vi "Measurement UI.vi"() -> ()   [LabVIEW 2021, in "Advanced Data Structure Exchange UI.lvlib"]
uses:
  Advanced Data Structure Exchange UI.lvlib
  Advanced Data Structure Exchange/Cluster In.ctl
  Advanced Data Structure Exchange/Cluster Out.ctl
  f0fe0f58-f2b4-4143-8e8a-3af1e57b7123.vi
  ddf3fbea-121e-4524-8916-c867006085d0.vi
  830132d3-c9aa-4633-b2df-af3633884cec.vi
  de374512-88bd-4d17-83f8-57bd328874a2.vi
  <vilib>/JDP Science/JSONtext/Variant to JSON Text.vi
  <vilib>/JDP Science/JSONtext/JSON text to Variant.vi
  <vilib>/JDP Science/JSONtext/LVClass Serializer/JSONtext LVClass Serializer.lvclass
  Advanced Data Structure Exchange/Advanced Data Structure Exchange.lvlib
panel:
  out "Cluster Out str":string
  in  "Cluster In str":string
  in  "Data Exchange Medium":enum32{"JSON String", "Text File"}(ring)
  in  "Text File Path":path
  out "Cluster Out":T1
  in  "Cluster In":T2 {"Text Ring" items=["Default", "Custom"]}
  # "(Choose only if Date exchange is through File)"
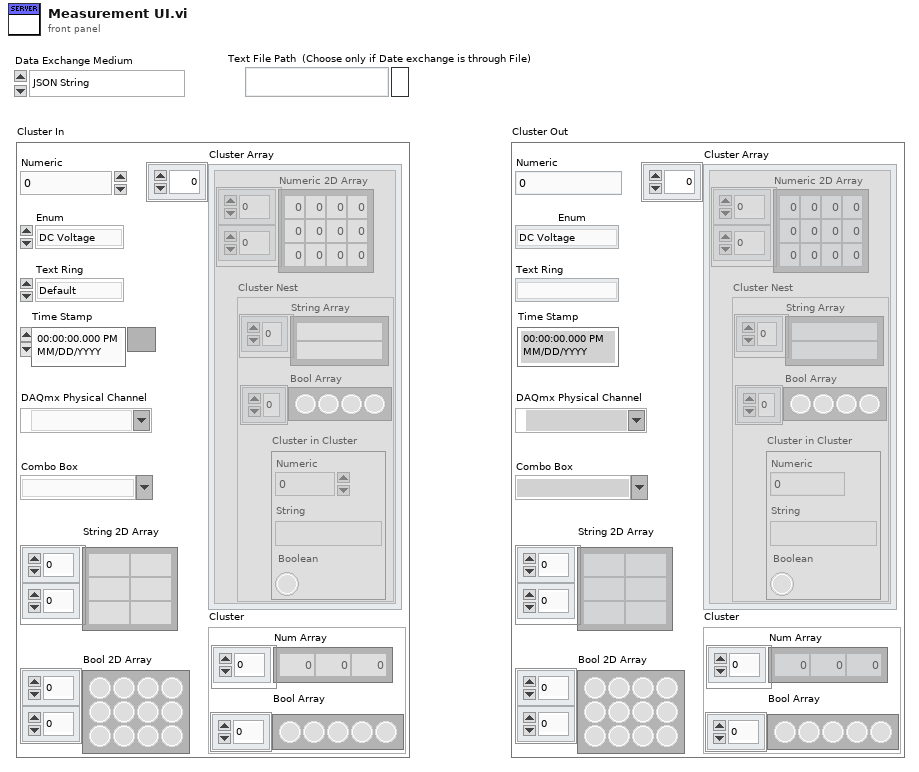
[diagram p1: front panel]
types:
  T1 = typedef "Advanced Data Structure Exchange.lvlib/Cluster Out.ctl" = cluster{"Numeric":dbl, "Bool 2D Array":bool[][], "String 2D Array":string[][], "Text Ring":u16, "Cluster":cluster{"Num Array":dbl[], "Bool Array":bool[]}, "Time Stamp":timestamp, "Enum":enum16{"DC Voltage", "DC Current"}, "DAQmx Physical Channel":tag, "Combo Box":string, "Cluster Array":cluster{"Numeric 2D Array":dbl[][], "Cluster Nest":cluster{"String Array":string[], "Bool Array":bool[], "Cluster in Cluster":cluster{"Numeric":dbl, "Boolean":bool, "String":string}}}[]}
  T2 = typedef "Advanced Data Structure Exchange.lvlib/Cluster In.ctl" = cluster{"Numeric":dbl, "Bool 2D Array":bool[][], "String 2D Array":string[][], "Text Ring":u16, "Cluster":cluster{"Num Array":dbl[], "Bool Array":bool[]}, "Time Stamp":timestamp, "Enum":enum16{"DC Voltage", "DC Current"}, "DAQmx Physical Channel":tag, "Combo Box":string, "Cluster Array":cluster{"Numeric 2D Array":dbl[][], "Cluster Nest":cluster{"String Array":string[], "Bool Array":bool[], "Cluster in Cluster":cluster{"Numeric":dbl, "Boolean":bool, "String":string}}}[]}
  T3 = enum16{"open", "replace", "create", "open or create", "replace or create", "replace or create with confirmation"}
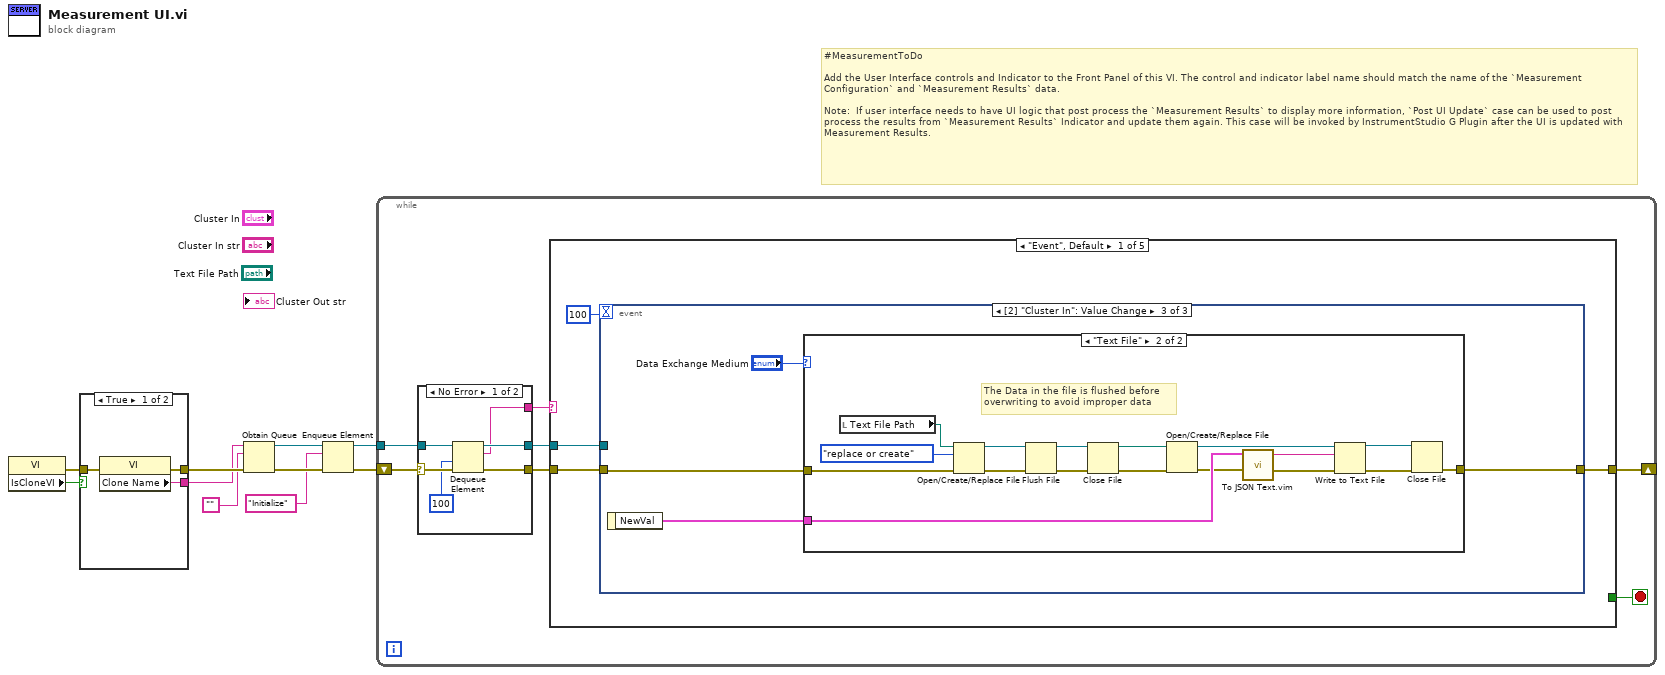
[diagram p0: block diagram]
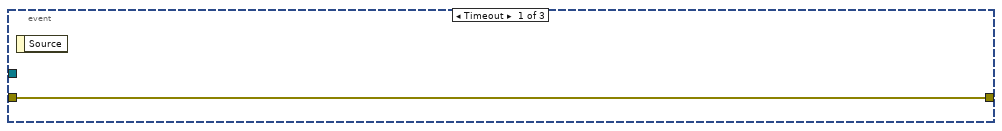
[diagram p2: hidden frame]
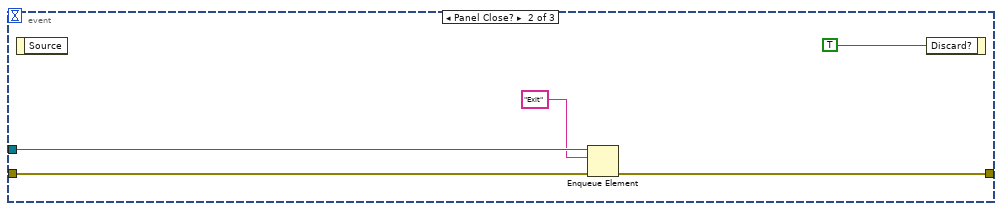
[diagram p3: hidden frame]
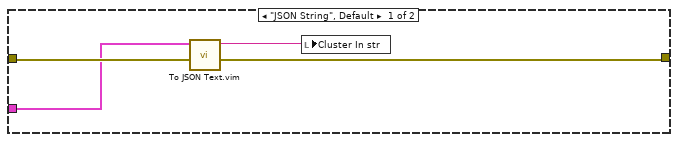
[diagram p4: hidden frame]
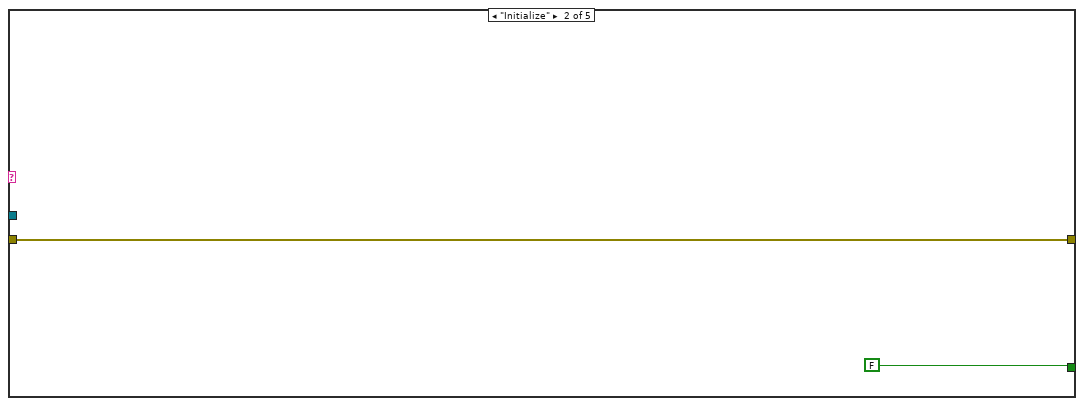
[diagram p5: hidden frame]
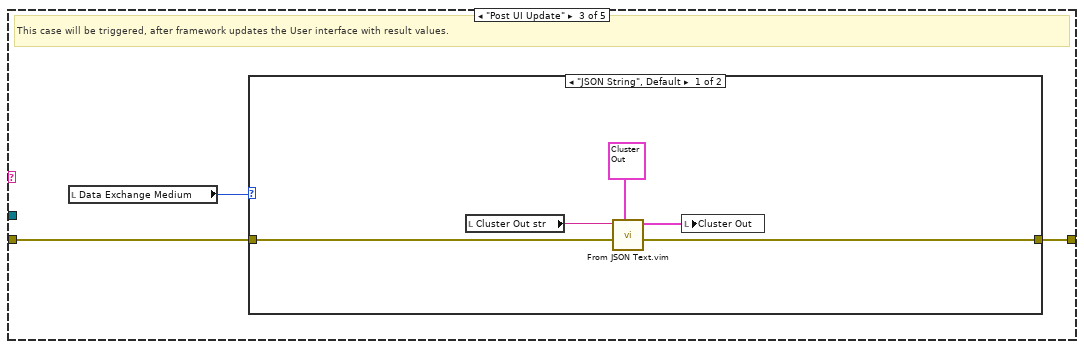
[diagram p6: hidden frame]
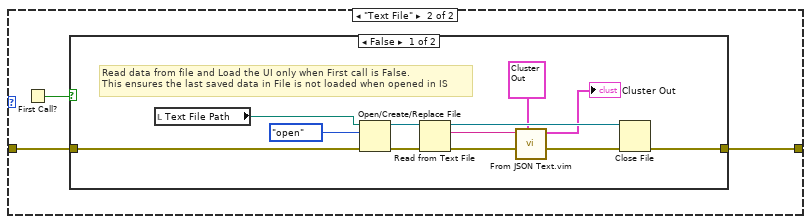
[diagram p7: hidden frame]
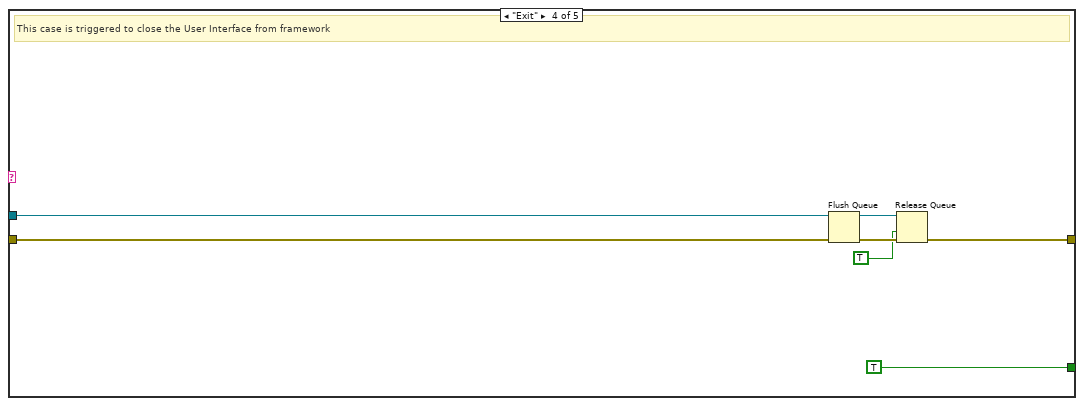
[diagram p9: hidden frame]
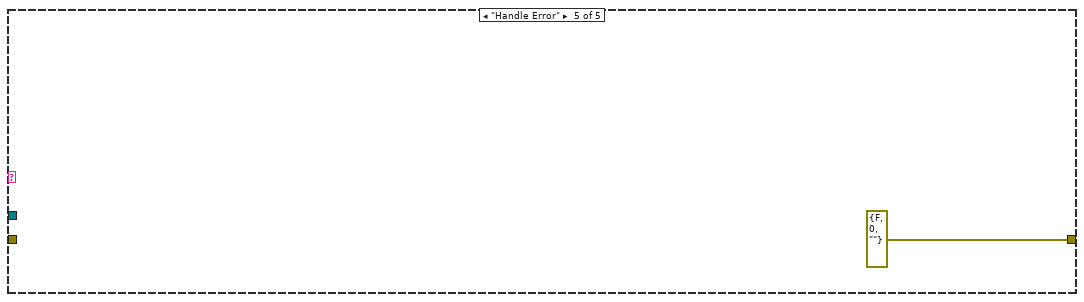
[diagram p10: hidden frame]
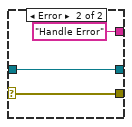
[diagram p11: hidden frame]
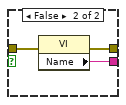
[diagram p12: hidden frame]
diagram:
  # "#MeasurementToDo  \n\nAdd the User Interface controls and Indicator to the Front Panel of this VI. The control and indicator label name should match the name of the `Measurement Configuration` and `Measurement Results` data.\n\nNote:  If user interface needs to have UI logic that post process the `Measurement Results` to display more information, `Post UI Update` case can be used to post process the results from `Measurement Results` Indicator and update them again. This case will be invoked by InstrumentStudio G Plugin after the UI is updated with Measurement Results."
  n1 = property class="VI"() -> (error out=w1:errorcluster, "IsCloneVI"=w2:bool)  [unwired: 2 in, 1 out]
  n2 = case shown="True" w2 {
    tunnel: [w13 w16] -> w10
    tunnel: [w12 w15] -> w9
    tunnel: w1 -> [w11 w14]
    frame True {
      n3 = property class="VI"(error in=w11) -> (error out=w13:errorcluster, "Clone Name"=w12:string)  [unwired: 1 in, 1 out]
    }
    frame False {
      n4 = property class="VI"(error in=w14) -> (error out=w16:errorcluster, "Name"=w15:string)  [unwired: 1 in, 1 out]
    }
  }
  n5 = Obtain Queue(name (unnamed)=w9, element data type="", error in (no error)=w10) -> (queue out=w6:refnum<queue>, error out=w8:errorcluster)  [unwired: 2 in, 1 out]
  n6 = Enqueue Element(queue=w6, element="Initialize", error in (no error)=w8) -> (queue out=w5:refnum<queue>, error out=w7:errorcluster)  [unwired: 1 in, 1 out]
  n7 = while {
    shift-right: [w18] -> _
    shift-left: w7 -> [w23]
    tunnel: w5 -> [w21]
    stop <- w17 stop-if-true
    n8 = case shown="No Error" w23 {
      selector: w23 -> [w98 w101]
      tunnel: [w97 w101] -> w22
      tunnel: w21 -> [w96 w100]
      tunnel: [w95 w100] -> w20
      tunnel: [w94 "Handle Error"] -> w19
      frame No Error {
        n9 = Dequeue Element(queue=w96, timeout in ms (-1)=100, error in (no error)=w98) -> (queue out=w95:refnum<queue>, element=w94:string, error out=w97:errorcluster)  [unwired: 1 out]
      }
      frame Error {
      }
    }
    n10 = case shown="\"Event\", Default" w19 {
      tunnel: w22 -> [w26 w60 w62 w91 _]
      tunnel: w20 -> [w24 _ _ w89 _]
      tunnel: [w27 w60 w63 w86 errorcluster {"status"=FALSE, "code"=0, "source"=""} ("error out")] -> w18
      tunnel: [_ FALSE _ TRUE _] -> w17
      frame "Event", Default {
        n11 = event shown="[2] \"Cluster In\": Value Change" {
          selector: _ -> [_ _ _]
          dyn-events: _ -> [_ _ _]
          timeout: 100 -> [_ _ _]
          tunnel: [w28 w31 w35] -> w27
          tunnel: w26 -> [w28 w32 w36]
          tunnel: w24 -> [_ w30 _]
          event Timeout {
            n12 = event-data() -> ()  [unwired: 1 in, 1 out]
          }
          event Panel Close? {
            n13 = event-data() -> ()  [unwired: 1 in, 1 out]
            n14 = Enqueue Element(queue=w30, element="Exit", error in (no error)=w32) -> (error out=w31:errorcluster)  [unwired: 1 in, 2 out]
            n15 = event-data("Discard?"=TRUE) -> ()  [unwired: 1 in, 1 out]
          }
          event Value Change {
            n16 = event-data() -> ("NewVal"=w37:T2)  [unwired: 1 in]
            n17 = case shown="\"Text File\"" "Data Exchange Medium" {
              tunnel: w37 -> [w40 w58]
              tunnel: w36 -> [w41 w50]
              tunnel: [w38 w43] -> w35
              frame "JSON String", Default {
                n18 = call "To JSON Text.vim"("error in (no error)"=w41, "Anything"=w40) -> ("error out"=w38:errorcluster, "<JSON>"=w39:string)  [unwired: 8 in]
                n19 = local write "Cluster In str"(w39) -> ()
              }
              frame "Text File" {
                # "The Data in the file is flushed before \noverwriting to avoid improper data"
                n20 = local read "Text File Path"() -> (w42:path)
                n21 = Open/Create/Replace File(file path (use dialog)=w42, error in=w50, operation (0:open)=T3."replace or create") -> (refnum out=w51:refnum<file>, error out=w48:errorcluster)  [unwired: 3 in, 1 out]
                n22 = Flush File(refnum=w51, error in=w48) -> (refnum out=w56:refnum<file>, error out=w47:errorcluster)
                n23 = Close File(refnum=w56, error in=w47) -> (path=w55:path, error out=w46:errorcluster)
                n24 = Open/Create/Replace File(file path (use dialog)=w55, error in=w46) -> (refnum out=w54:refnum<file>, error out=w49:errorcluster)  [unwired: 4 in, 1 out]
                n25 = call "To JSON Text.vim"("error in (no error)"=w49, "Anything"=w58) -> ("error out"=w45:errorcluster, "<JSON>"=w57:string)  [unwired: 8 in]
                n26 = Write to Text File(file (use dialog)=w54, text=w57, error in=w45) -> (refnum out=w53:refnum<file>, error out=w44:errorcluster)  [unwired: 1 in, 1 out]
                n27 = Close File(refnum=w53, error in=w44) -> (error out=w43:errorcluster)  [unwired: 1 out]
              }
            }
          }
        }
      }
      frame "Initialize" {
      }
      frame "Post UI Update" {
        # "This case will be triggered, after framework updates the User interface with result values."
        n28 = local read "Data Exchange Medium"() -> (w61:enum32{"JSON String", "Text File"})
        n29 = case shown="\"JSON String\", Default" w61 {
          tunnel: [w67 w71] -> w63
          tunnel: w62 -> [w68 w70]
          frame "JSON String", Default {
            n30 = local read "Cluster Out str"() -> (w66:string)
            n31 = call "From JSON Text.vim"("Data Type and Default Value"=T1 {"Numeric"=0.0, "Bool 2D Array"=[], "String 2D Array"=[], "Text Ring"=0, "Cluster"={"Num Array"=[], "Bool Array"=[]}, "Time Stamp"=timestamp(0 s since 1904-01-01), "Enum"=enum."DC Voltage", "DAQmx Physical Channel"="", "Combo Box"="", "Cluster Array"=[]} ("Cluster Out"), "error in (no error)"=w68, "JSON"=w66) -> ("error out"=w67:errorcluster, "Data out"=w64:T1)  [unwired: 7 in]
            n32 = local write "Cluster Out"(w64) -> ()
          }
          frame "Text File" {
            n33 = First Call?() -> (First Call?: T/F=w69:bool)
            n34 = case shown="False" w69 {
              tunnel: [w83 w84] -> w71
              tunnel: w70 -> [w82 w84]
              frame False {
                # "Read data from file and Load the UI only when First call is False.\nThis ensures the last saved data in File is not loaded when opened in IS"
                n35 = local read "Text File Path"() -> (w72:path)
                n36 = Open/Create/Replace File(file path (use dialog)=w72, error in=w82, operation (0:open)=T3."open") -> (refnum out=w81:refnum<file>, error out=w78:errorcluster)  [unwired: 3 in, 1 out]
                n37 = Read from Text File(file (use dialog)=w81, error in=w78) -> (refnum out=w80:refnum<file>, text=w75:string, error out=w74:errorcluster)  [unwired: 2 in, 1 out]
                n38 = call "From JSON Text.vim"("Data Type and Default Value"=T1 {"Numeric"=0.0, "Bool 2D Array"=[], "String 2D Array"=[], "Text Ring"=0, "Cluster"={"Num Array"=[], "Bool Array"=[]}, "Time Stamp"=timestamp(0 s since 1904-01-01), "Enum"=enum."DC Voltage", "DAQmx Physical Channel"="", "Combo Box"="", "Cluster Array"=[]} ("Cluster Out"), "error in (no error)"=w74, "JSON"=w75) -> ("error out"=w79:errorcluster, "Data out"=→"Cluster Out":T1)  [unwired: 7 in]
                n39 = Close File(refnum=w80, error in=w79) -> (error out=w83:errorcluster)  [unwired: 1 out]
              }
              frame True {
              }
            }
          }
        }
      }
      frame "Exit" {
        # "This case is triggered to close the User Interface from framework"
        n40 = Flush Queue(queue=w89, error in (no error)=w91) -> (queue out=w88:refnum<queue>, error out=w87:errorcluster)  [unwired: 1 out]
        n41 = Release Queue(queue=w88, force destroy? (F)=TRUE, error in (no error)=w87) -> (error out=w86:errorcluster)  [unwired: 2 out]
      }
      frame "Handle Error" {
      }
    }
  }
